vi "LabVIEW file.vi"() -> ()   [LabVIEW 2022 SP3]
uses:
  <vilib>/DAQmx/write.llb/DAQmx Write (Digital Bool 1Line 1Point).vi
  <vilib>/DAQmx/read.llb/DAQmx Read (Digital Bool 1Line 1Point).vi
  <vilib>/DAQmx/read.llb/DAQmx Read (Analog DBL 1Chan 1Samp).vi
  <vilib>/DAQmx/write.llb/DAQmx Write (Digital U8 1Chan 1Samp).vi
  <vilib>/DAQmx/create/channels.llb/DAQmx Create Channel (DO-Digital Output).vi
  <vilib>/DAQmx/create/channels.llb/DAQmx Create Channel (AI-Voltage-Basic).vi
  <vilib>/DAQmx/miscellaneous.llb/DAQmx Fill In Error Info.vi
  <vilib>/DAQmx/create/channels.llb/DAQmx Create Channel (DI-Digital Input).vi
  <vilib>/Instr/_visa.llb/VISA Configure Serial Port (Instr).vi
  <vilib>/httpClient/PUTBuffer.vi
  <vilib>/httpClient/LabVIEWHTTPClient.lvlib
panel:
  out "Humidity":dbl
  out "Temperature":dbl
  out "Soil Moisture":dbl
  in  "Enable Termination\nChar (T)":bool=TRUE
  in  "VISA resource name":refnum<visa-resource-name>
  in  "Website Data Stop":bool
  in  "Water Pump Output":tag
  in  "Buzzer Output":tag
  in  "Rain Sensor Input":tag
  out "Rain Indicator":bool
  in  "stop 2":bool
  in  "Irrigation Control":bool
  out "Irriggation System":bool
  in  "Match Status":bool
  out "SoilMoisture":dbl(knob) scale=0.0..100.0
  out "Temperature":dbl(slide) scale=0.0..100.0
  out "Humidity":dbl(knob) scale=0.0..100.0
  in  "lux_voltage_input":tag
  in  "relay_input":tag
  in  "stop":bool
  out "Stage  1":bool
  out "Active Light Stages":dbl
  out "Stage 2":bool
  out "Stage 3":bool
  out "Stage  4":bool
  out "Lux Reading":dbl
  out "Lux Meter":dbl(knob) scale=0.0..800.0
  in  "Stage 1":bool
  in  "Stage 2":bool
  in  "Stage 3":bool
  in  "Stage 4":bool
  in  "Manual or Automatic Lighting Control":bool
  out "Flood Lights Indicator":bool
  # "Automated Cricket Ground Control System"
  # "DAQ Ports"
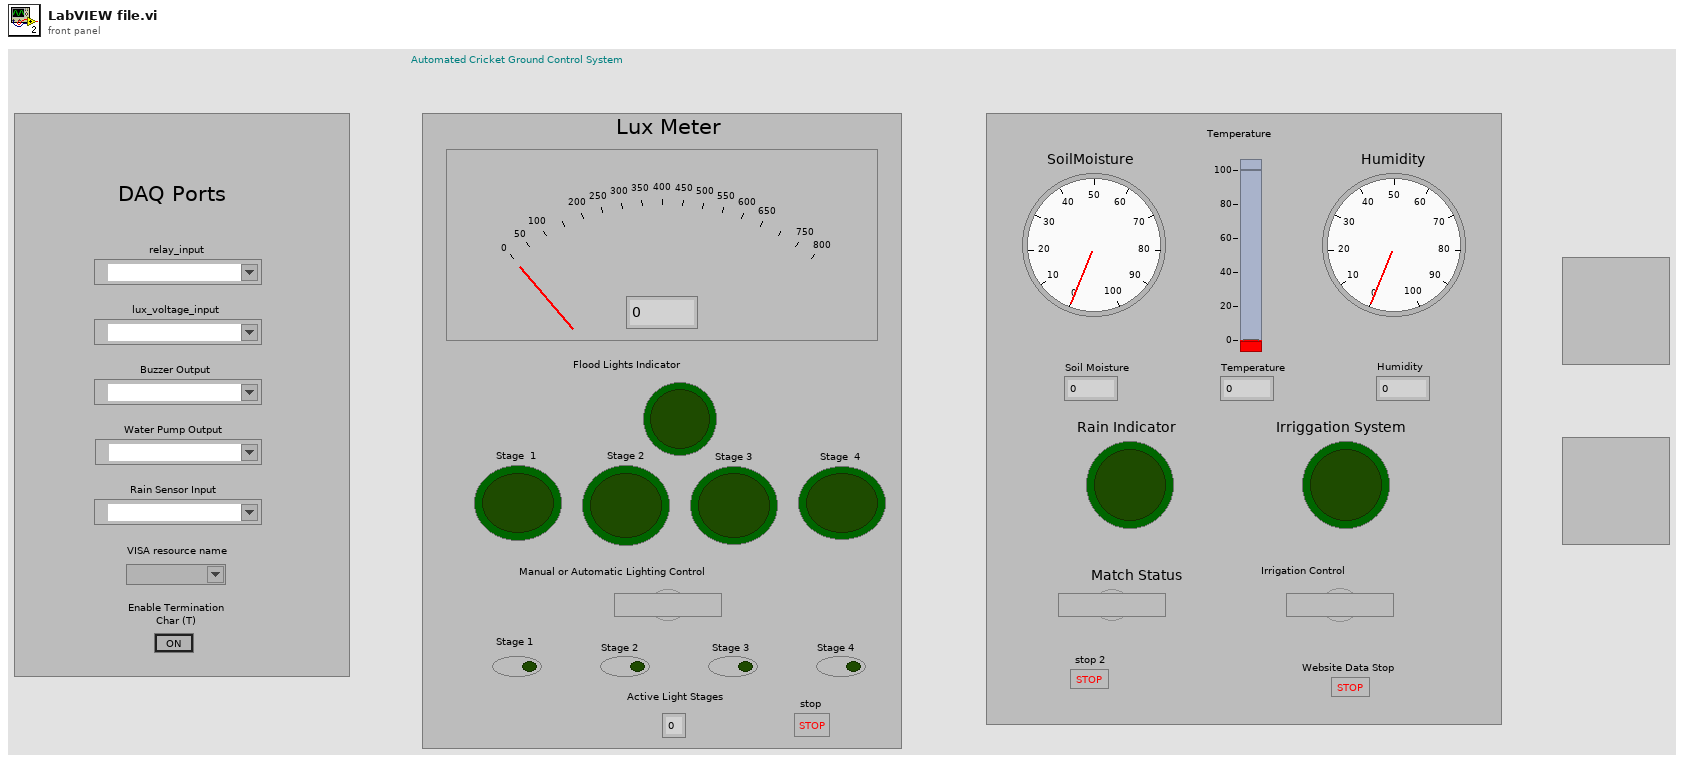
[diagram p1: front panel]
types:
  T1 = typedef "LabVIEWHTTPClient.lvlib/ClientHandle.ctl" = refnum<k1>
  T2 = cluster{"rain":bool, "soilMoisture":i32, "matchStatus":bool, "floodLights":bool, "irrigation":bool, "drainagePump":bool, "lastUpdated":string, "light":dbl, "temperature":dbl, "humidity":dbl}
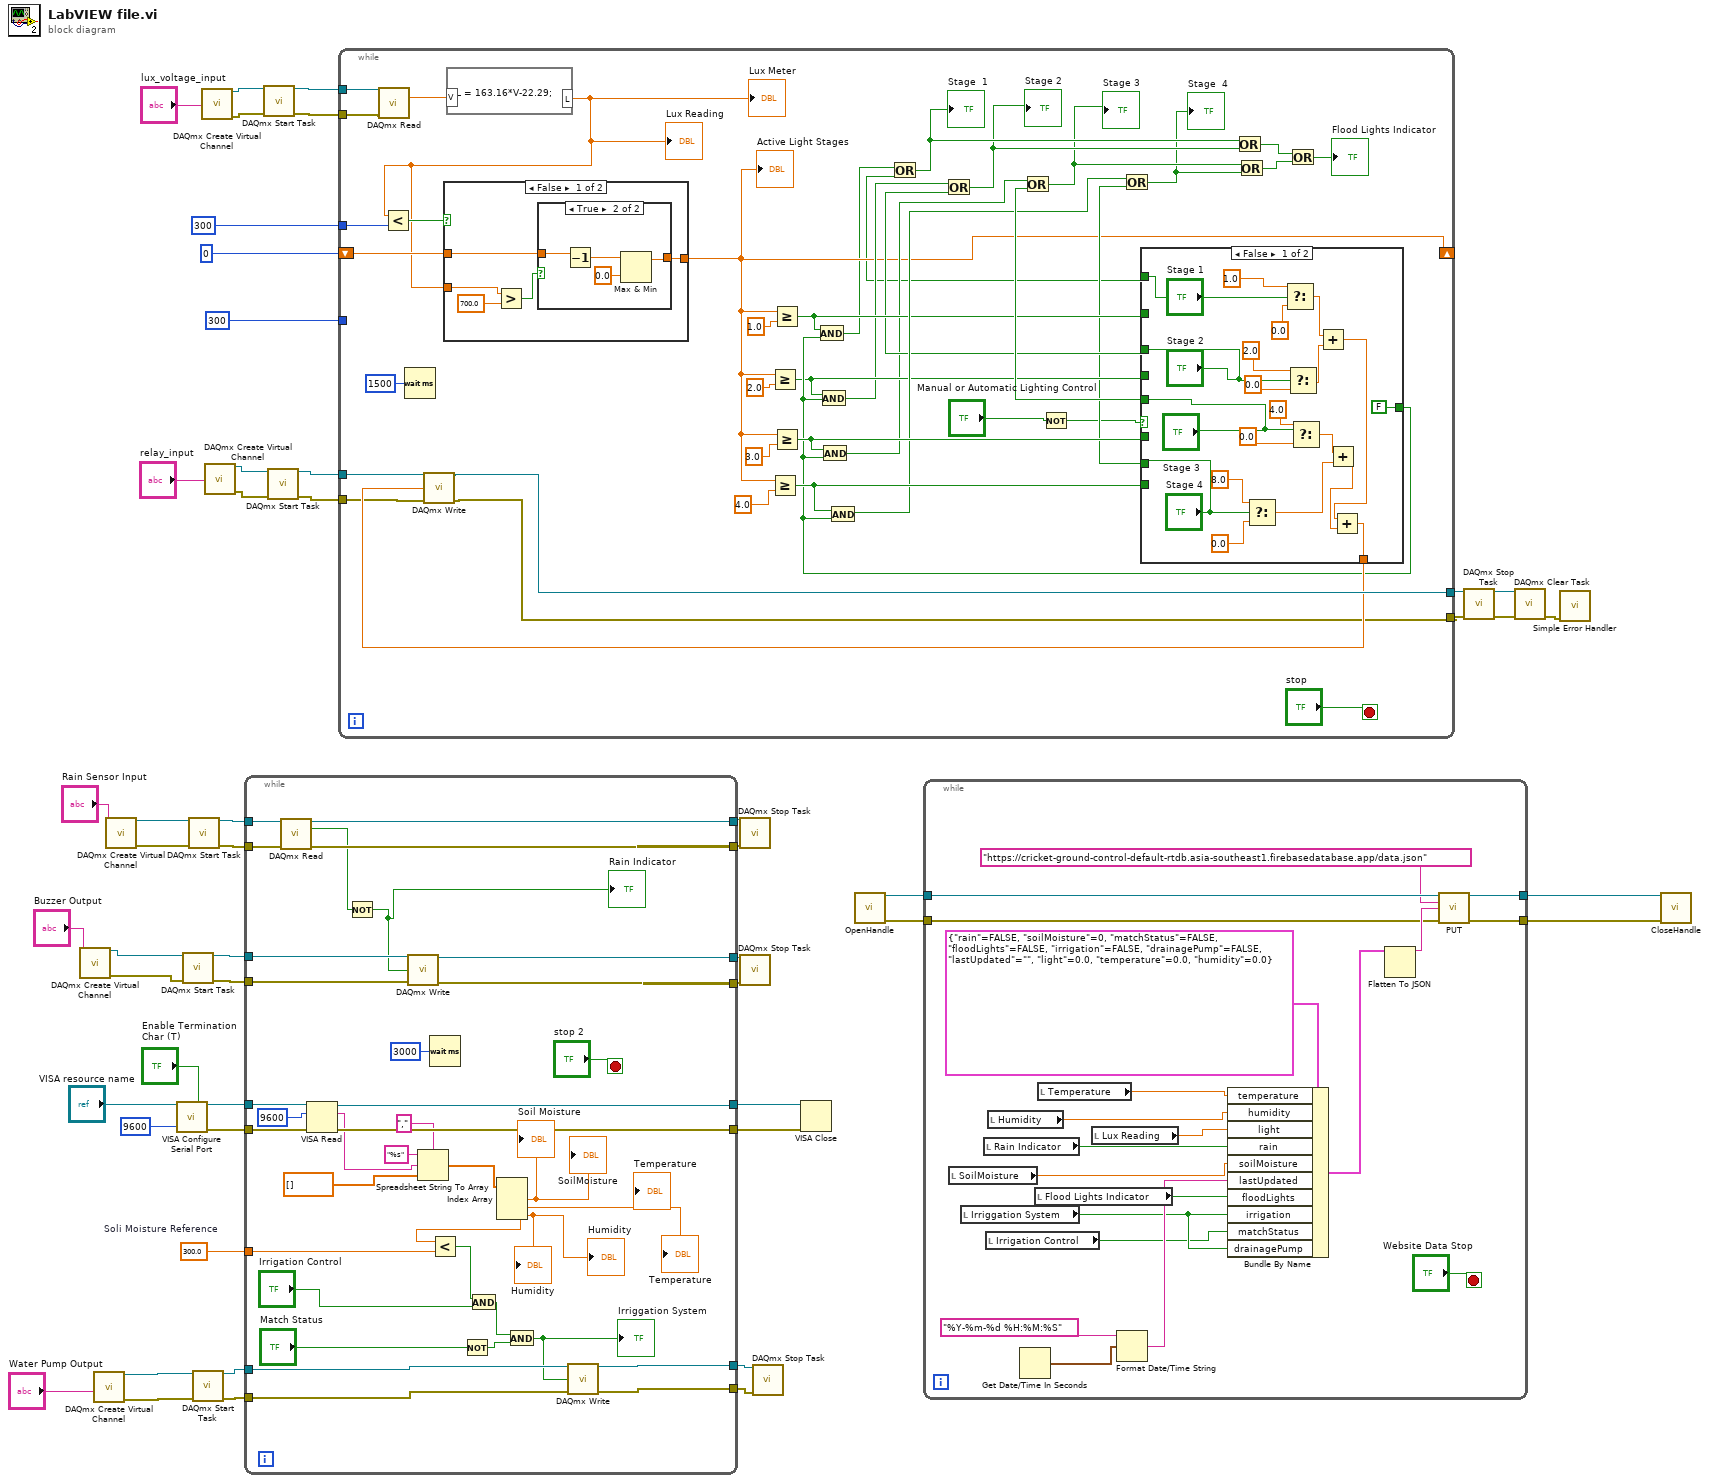
[diagram p0: block diagram]
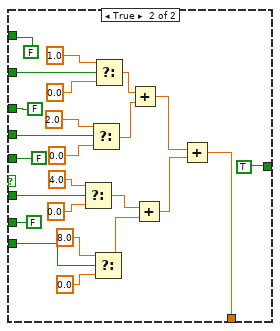
[diagram p2: hidden frame]
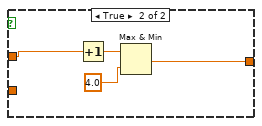
[diagram p4: hidden frame]
diagram:
  w1 = 300.0  # Soli Moisture Reference
  n1 = call-poly <vilib>:"DAQmx Create Virtual Channel.vi"("lines"="Buzzer Output") -> ("task out"=w25:refnum<k21>, "error out"=w24:errorcluster)  [unwired: 13 in]
  n2 = call-poly <vilib>:"DAQmx Create Virtual Channel.vi"("lines"="Water Pump Output") -> ("task out"=w14:refnum<k21>, "error out"=w13:errorcluster)  [unwired: 13 in]
  n3 = call-poly <vilib>:"DAQmx Create Virtual Channel.vi"("lines"="Rain Sensor Input") -> ("task out"=w32:refnum<k21>, "error out"=w31:errorcluster)  [unwired: 13 in]
  n4 = call-poly "VISA Configure Serial Port"("VISA resource name"="VISA resource name", "Enable Termination\nChar (T)"="Enable Termination\nChar (T)", "baud rate (9600)"=u32 9600) -> ("VISA resource name out"=w18:refnum<visa-resource-name>, "error out"=w17:errorcluster)  [unwired: 11 in]
  n5 = call <vilib>:"DAQmx Start Task.vi"("task/channels in"=w25, "error in"=w24) -> ("task out"=w23:refnum<k21>, "error out"=w22:errorcluster)  [unwired: 12 in]
  n6 = call <vilib>:"DAQmx Start Task.vi"("task/channels in"=w32, "error in"=w31) -> ("task out"=w30:refnum<k21>, "error out"=w29:errorcluster)  [unwired: 12 in]
  n7 = call <vilib>:"DAQmx Start Task.vi"("task/channels in"=w14, "error in"=w13) -> ("task out"=w11:refnum<k21>, "error out"=w10:errorcluster)  [unwired: 12 in]
  n8 = call-poly <vilib>:"DAQmx Create Virtual Channel.vi"("physical channels"="lux_voltage_input") -> ("task out"=w38:refnum<k21>, "error out"=w37:errorcluster)  [unwired: 13 in]
  n9 = call-poly <vilib>:"DAQmx Create Virtual Channel.vi"("lines"="relay_input") -> ("task out"=w45:refnum<k21>, "error out"=w47:errorcluster)  [unwired: 13 in]
  n10 = while {
    tunnel: w30 -> [w87]
    tunnel: w29 -> [w86]
    tunnel: [w85] -> w28
    tunnel: [w84] -> w27
    tunnel: w23 -> [w82]
    tunnel: w22 -> [w81]
    tunnel: [w80] -> w21
    tunnel: [w79] -> w20
    tunnel: w11 -> [w73]
    tunnel: w10 -> [w72]
    tunnel: [w71] -> w9
    tunnel: [w70] -> w8
    tunnel: w18 -> [w77]
    tunnel: [w75] -> w16
    tunnel: w17 -> [w76]
    tunnel: [w74] -> w15
    tunnel: w1 -> [w53]
    stop <- "stop 2" stop-if-true
    n11 = call-poly <vilib>:"DAQmx Read.vi"("task/channels in"=w87, "error in"=w86) -> ("task out"=w85:refnum<k21>, "data"=w67:bool, "error out"=w84:errorcluster)  [unwired: 11 in]
    n12 = VISA Read(VISA resource name=w77, byte count=u32 9600, error in (no error)=w76) -> (VISA resource name out=w75:refnum<visa-resource-name>, read buffer=w61:string, error out=w74:errorcluster)  [unwired: 1 out]
    n13 = Not(x=w67) -> (.not. x?=w52:bool)
    "Rain Indicator" <- w52
    n14 = call-poly <vilib>:"DAQmx Write.vi"("task/channels in"=w82, "data"=w52, "error in"=w81) -> ("task out"=w80:refnum<k21>, "error out"=w79:errorcluster)  [unwired: 10 in, 1 out]
    n15 = Spreadsheet String To Array(delimiter (Tab)=",", format string="%s", spreadsheet string=w61, array type (2D Dbl)=dbl[] []) -> (array=w57:dbl[])
    n16 = Wait (ms)(milliseconds to wait=u32 3000) -> ()  [unwired: 1 out]
    n17 = Not(x="Match Status") -> (.not. x?=w64:bool)
    n18 = Index Array(array=w57) -> (element #1=w54:dbl, element #2=→"Temperature" →"Temperature":dbl, element #3=→"Humidity" →"Humidity":dbl)  [unwired: 3 in]
    "SoilMoisture" <- w54
    "Soil Moisture" <- w54
    n19 = Less?(x=w54, y=w53) -> (x < y?=w69:bool)
    n20 = And(x=w69, y="Irrigation Control") -> (x .and. y?=w63:bool)
    n21 = And(x=w63, y=w64) -> (x .and. y?=w62:bool)
    "Irriggation System" <- w62
    n22 = call-poly <vilib>:"DAQmx Write.vi"("task/channels in"=w73, "data"=w62, "error in"=w72) -> ("task out"=w71:refnum<k21>, "error out"=w70:errorcluster)  [unwired: 10 in, 1 out]
  }
  n23 = call <vilib>:"DAQmx Start Task.vi"("task/channels in"=w38, "error in"=w37) -> ("task out"=w35:refnum<k21>, "error out"=w36:errorcluster)  [unwired: 12 in]
  n24 = call <vilib>:"DAQmx Start Task.vi"("task/channels in"=w45, "error in"=w47) -> ("task out"=w44:refnum<k21>, "error out"=w46:errorcluster)  [unwired: 12 in]
  n25 = while {
    shift-right: [w101] -> _
    shift-left: 0 -> [w124]
    tunnel: 300 -> [w128]
    tunnel: 300 -> [_]
    tunnel: w46 -> [w111]
    tunnel: w44 -> [w120]
    tunnel: [w119] -> w43
    tunnel: [w102] -> w42
    tunnel: w36 -> [w116]
    tunnel: w35 -> [w118]
    stop <- "stop" stop-if-true
    n26 = call-poly <vilib>:"DAQmx Read.vi"("task/channels in"=w118, "error in"=w116) -> ("data"=w117:dbl)  [unwired: 11 in, 2 out]
    n27 = Wait (ms)(milliseconds to wait=u32 1500) -> ()  [unwired: 1 out]
    n28 = formula code="L = 163.16*V-22.29;"("V"=w117) -> ("L"=w98:dbl)
    "Lux Reading" <- w98
    "Lux Meter" <- w98
    n29 = Less?(x=w98, y=w128) -> (x < y?=w127:bool)
    n30 = case shown="False" w127 {
      tunnel: [w173 w183] -> w101
      tunnel: w124 -> [w174 w184]
      tunnel: w98 -> [w176 _]
      frame False {
        n31 = Greater?(x=w176, y=700.0) -> (0:w175:bool)
        n32 = case shown="True" w175 {
          tunnel: w174 -> [w178 w182]
          tunnel: [w178 w179] -> w173
          frame False {
          }
          frame True {
            n33 = Decrement(x=w182) -> (x-1=w181:dbl)
            n34 = Max & Min(x=w181, y=0.0) -> (max(x,y)=w179:dbl)  [unwired: 1 out]
          }
        }
      }
      frame True {
        n35 = Increment(x=w184) -> (x+1=w186:dbl)
        n36 = Max & Min(x=w186, y=4.0) -> (min(x,y)=w183:dbl)  [unwired: 1 out]
      }
    }
    "Active Light Stages" <- w101
    n37 = Greater Or Equal?(x=w101, y=2.0) -> (x >= y?=w107:bool)
    n38 = Greater Or Equal?(x=w101, y=4.0) -> (x >= y?=w113:bool)
    n39 = Greater Or Equal?(x=w101, y=1.0) -> (x >= y?=w108:bool)
    n40 = Greater Or Equal?(x=w101, y=3.0) -> (x >= y?=w114:bool)
    n41 = Not(x="Manual or Automatic Lighting Control") -> (.not. x?=w88:bool)
    n42 = case shown="False" w88 {
      tunnel: w108 -> [_ w172]
      tunnel: w107 -> [_ w171]
      tunnel: w114 -> [_ w170]
      tunnel: w113 -> [_ w169]
      tunnel: [w136 w155] -> w112
      tunnel: ["Stage 1" FALSE ("s")] -> w90
      tunnel: ["Stage 2" FALSE ("s 2")] -> w106
      tunnel: ["Stage 3" FALSE ("s 3")] -> w115
      tunnel: ["Stage 4" FALSE ("s 4")] -> w103
      tunnel: [FALSE TRUE] -> w109
      frame False {
        n43 = Select(t=8.0, s="Stage 4", f=0.0) -> (s? t:f=w146:dbl)
        n44 = Select(t=1.0 ("s? t:f"), s="Stage 1", f=0.0) -> (s? t:f=w144:dbl)
        n45 = Select(t=2.0, s="Stage 2", f=0.0) -> (s? t:f=w145:dbl)
        n46 = Select(t=4.0, s="Stage 3", f=0.0) -> (s? t:f=w147:dbl)
        n47 = Add(x=w144, y=w145) -> (x+y=w130:dbl)
        n48 = Add(x=w147, y=w146) -> (x+y=w148:dbl)
        n49 = Add(x=w130, y=w148) -> (x+y=w136:dbl)
      }
      frame True {
        n50 = Select(t=4.0, s=w170, f=0.0) -> (s? t:f=w157:dbl)
        n51 = Select(t=2.0, s=w171, f=0.0) -> (s? t:f=w159:dbl)
        n52 = Select(t=8.0, s=w169, f=0.0) -> (s? t:f=w158:dbl)
        n53 = Select(t=1.0 ("s? t:f"), s=w172, f=0.0) -> (s? t:f=w160:dbl)
        n54 = Add(x=w160, y=w159) -> (x+y=w150:dbl)
        n55 = Add(x=w157, y=w158) -> (x+y=w156:dbl)
        n56 = Add(x=w150, y=w156) -> (x+y=w155:dbl)
      }
    }
    n57 = call-poly <vilib>:"DAQmx Write.vi"("task/channels in"=w120, "data"=w112, "error in"=w111) -> ("task out"=w119:refnum<k21>, "error out"=w102:errorcluster)  [unwired: 10 in, 1 out]
    n58 = And(x=w108, y=w109) -> (x .and. y?=w100:bool)
    n59 = And(x=w107, y=w109) -> (x .and. y?=w105:bool)
    n60 = And(x=w114, y=w109) -> (x .and. y?=w104:bool)
    n61 = And(x=w113, y=w109) -> (x .and. y?=w110:bool)
    n62 = Or(x=w100, y=w90) -> (x .or. y?=w95:bool)
    "Stage  1" <- w95
    n63 = Or(x=w105, y=w106) -> (x .or. y?=w94:bool)
    "Stage 2" <- w94
    n64 = Or(x=w104, y=w115) -> (x .or. y?=w93:bool)
    "Stage 3" <- w93
    n65 = Or(x=w110, y=w103) -> (x .or. y?=w92:bool)
    "Stage  4" <- w92
    n66 = Or(x=w95, y=w94) -> (x .or. y?=w97:bool)
    n67 = Or(x=w93, y=w92) -> (x .or. y?=w96:bool)
    n68 = Or(x=w97, y=w96) -> (x .or. y?=→"Flood Lights Indicator":bool)
  }
  n69 = call <vilib>:"DAQmx Stop Task.vi"("task/channels in"=w28, "error in"=w27) -> ()  [unwired: 12 in, 2 out]
  n70 = call <vilib>:"DAQmx Stop Task.vi"("task/channels in"=w21, "error in"=w20) -> ()  [unwired: 12 in, 2 out]
  n71 = call <vilib>:"DAQmx Stop Task.vi"("task/channels in"=w9, "error in"=w8) -> ()  [unwired: 12 in, 2 out]
  n72 = VISA Close(VISA resource name=w16, error in (no error)=w15) -> ()  [unwired: 1 out]
  n73 = call <vilib>:"OpenHandle.vi"() -> ("client handle out"=w7:T1, "error out"=w6:errorcluster)  [unwired: 14 in]
  n74 = while {
    tunnel: w7 -> [w205]
    tunnel: w6 -> [w204]
    tunnel: [w202] -> w5
    tunnel: [w201] -> w4
    stop <- "Website Data Stop" stop-if-true
    n75 = local read "SoilMoisture"() -> (w190:dbl)
    n76 = local read "Irriggation System"() -> (w192:bool)
    n77 = local read "Rain Indicator"() -> (w194:bool)
    n78 = local read "Irrigation Control"() -> (w191:bool)
    n79 = local read "Humidity"() -> (w187:dbl)
    n80 = Get Date/Time In Seconds() -> (seconds since 1Jan1904=w197:timestamp)
    n81 = local read "Flood Lights Indicator"() -> (w193:bool)
    n82 = local read "Temperature"() -> (w188:dbl)
    n83 = local read "Lux Reading"() -> (w189:dbl)
    n84 = Format Date/Time String(time format string (%c)="%Y-%m-%d %H:%M:%S", seconds (now)=w197) -> (date/time string=w195:string)  [unwired: 1 in]
    n85 = Bundle By Name(cluster=T2 {"rain"=FALSE, "soilMoisture"=0, "matchStatus"=FALSE, "floodLights"=FALSE, "irrigation"=FALSE, "drainagePump"=FALSE, "lastUpdated"="", "light"=0.0, "temperature"=0.0, "humidity"=0.0}, "temperature"=w188, "humidity"=w187, "light"=w189, "rain"=w194, "soilMoisture"=w190, "lastUpdated"=w195, "floodLights"=w193, "irrigation"=w192, "matchStatus"=w191, "drainagePump"=w192) -> (w198:T2)
    n86 = Flatten To JSON(anything=w198) -> (JSON string=w206:string)  [unwired: 2 in, 1 out]
    n87 = call-poly <vilib>:"PUT.vi"("client handle"=w205, "url"="https://cricket-ground-control-default-rtdb.asia-southeast1.firebasedatabase.app/data.json", "buffer"=w206, "error in (no error)"=w204) -> ("client handle out"=w202:T1, "error out"=w201:errorcluster)  [unwired: 8 in, 2 out]
  }
  n88 = call <vilib>:"DAQmx Stop Task.vi"("task/channels in"=w43, "error in"=w42) -> ("task out"=w39:refnum<k21>, "error out"=w41:errorcluster)  [unwired: 12 in]
  n89 = call <vilib>:"DAQmx Clear Task.vi"("task in"=w39, "error in"=w41) -> ("error out"=w40:errorcluster)  [unwired: 13 in]
  n90 = call <vilib>:"Simple Error Handler.vi"("error in (no error)"=w40) -> ()  [unwired: 4 in, 5 out]
  n91 = call <vilib>:"CloseHandle.vi"("client handle"=w5, "error in (no error)"=w4) -> ()  [unwired: 13 in, 1 out]
